vi "Process.vi"(8 "error in":errorcluster, 11 "Edit.Rect":refnum<class "Edit.Rect.lvclass">) -> (0 "error out":errorcluster, 3 "Edit.Rect out":refnum<class "Edit.Rect.lvclass">)   [LabVIEW 2019, in "Edit.Rect.lvclass"]
doc: "---------------------------------------------------------------\nJKI State Machine Objects™\nhttp://jki.net/state-machine-objects/\nCopyright (C) 2005-2015, JKI <info@jki.net>\nALL RIGHTS RESERVED"
uses:
  Edit.Rect.lvclass
  <vilib>/JKI/JKI SMO/SMO/SMO.lvclass
  <vilib>/JKI/JKI SMO/SMO/Typedefs/Parent Call--Enum.ctl
  Edit/Edit.lvclass
  subVIs/typedefs/Schedule Types/Schedule--Constant.ctl
  Settings/ObjectSettings/ObjectSettings.lvclass
  Settings/Setting Database/Setting Database.lvclass
  Settings/Rectangle Settings/Rectangle Settings.lvclass
  Settings/Setting Database/Typedefs/PrivateEvents--Setting Database.SetDefaultRectangle.ctl
  Settings/Setting Database/Typedefs/PrivateEvents--Setting Database.CopyActiveRectangleToAll.ctl
  C:/Users/Albro/Documents/GitHub/AFM-Lithography/lvsrc/Classes/Settings/ObjectSettings/ObjectSettings.lvclass
  C:/Program Files (x86)/National Instruments/LabVIEW 2019/vi.lib/JKI/JKI SMO/SMO/SMO.lvclass
  <vilib>/Utility/miscctls.llb/LVPointTypeDef.ctl
  Settings/Setting Database/Typedefs/PrivateEvents--Setting Database.Copy Settings To Group.ctl
panel:
  in  "Apply":bool
  out "Group String":string
  out "ID String":string
  in  "Apply All":bool
  in  "Speed Settings":bool
  in  "Voltage Settings":bool
  in  "Save Default":bool
  in  "Copy to All":bool
  in  "Fill Orientation":u16(ring) caption="Ring" items=["Horizontal", "Vertical"]
  in  "Enabled?":bool=TRUE
  in  "Direction":u16(ring) caption="Ring" items=["Forward", "Backward"]
  in  "Voltage Schedule":u16(ring) caption="Ring" items=["Constant", "Ramp", "Fn. Generator", "Formula"]
  in  "Speed Schedule":u16(ring) caption="Ring" items=["Constant", "Ramp", "Fn. Generator", "Formula"]
  in  "Set Resistance":T1(ring) caption="Enum"
  in  "Speed (um/s)":dbl caption="Numeric 2"
  in  "Voltage (V)":dbl caption="Numeric 2"
  in  "Fill Spacing":dbl caption="Numeric 2"
  # "For instructions on how to use the JKI State Machine Objects, examples and video tutorials, visit:\nhttp://jki.net/state-machine-objects/\n\nJKI State Machine Objects™\nhttp://jki.net/state-machine-objects/\nCopyright (C) 2005-2015, JKI <info@jki.net>\nALL RIGHTS RESERVED"
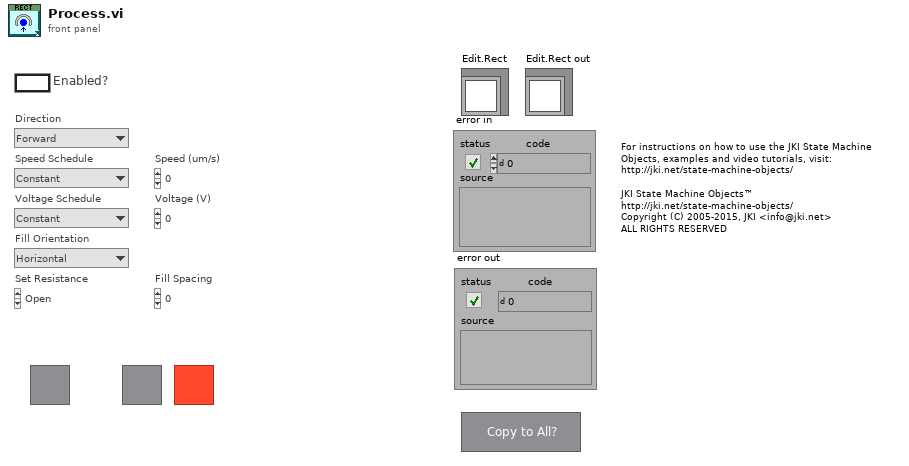
[diagram p1: front panel]
types:
  T1 = enum16{"Open", "Discharge Tip", "0 ohm", "100 kohm", "10 Mohm", "1 Gohm"}
  T2 = typedef "SMO.lvclass/Parent Call--Enum.ctl" = enum16{"Allows parent to run", "Does not request parent to run"}
  T3 = typedef "Schedule--Constant.ctl" = cluster{"Value":dbl}
  T4 = enum32{"invalid app kind", "Development System", "Run Time System", "Student Edition", "Embedded LabVIEW", "Evaluation", "Custom"}
  T5 = typedef "LVPointTypeDef.ctl" = cluster{"Horizontal":i16, "Vertical":i16}
  T6 = enum8{"Enabled", "Disabled", "Disabled and Grayed Out"}
  T7 = enum32{"Invalid", "Standard", "Closed", "Hidden", "Minimized", "Maximized"}
  T8 = enum32{"Bad", "Idle", "Run top level", "Running"}
  T9 = typedef "Setting Database.lvclass/PrivateEvents--Setting Database.Copy Settings To Group.ctl" = cluster{"Name":string, "Group":string}
  T10 = typedef "Setting Database.lvclass/PrivateEvents--Setting Database.SetDefaultRectangle.ctl" = bool
  T11 = typedef "Setting Database.lvclass/PrivateEvents--Setting Database.CopyActiveRectangleToAll.ctl" = bool
  T12 = typedef "Setting Database.lvclass/PublicEvents--Setting Database.NewActiveRectangle.ctl" = refnum<class "Rectangle Settings.lvclass">
  T13 = cluster{"Core":cluster{"Current VI Reference":refnum<vi>, "Close Panel on Exit?":bool, "error":errorcluster}, "Self":refnum<class "Edit.Rect.lvclass">, "SettingDB":refnum<class "Setting Database.lvclass">, "Rectangle Settings":refnum<class "Rectangle Settings.lvclass">}
  T14 = cluster{"Current VI Reference":refnum<vi>, "Close Panel on Exit?":bool, "error":errorcluster}
  T15 = enum16{"Always On", "Always Off", "Off While Running"}
  T16 = typedef "SMO.lvclass/Protected Events.ctl" = cluster{"StopProcesses":refnum<user-event>, "AbortProcesses":refnum<user-event>, "Config Changed":refnum<user-event>, "Dependency":refnum<user-event>}
  T17 = typedef "Setting Database.lvclass/PublicEvents--Cluster.ctl" = cluster{"NewActivePath":refnum<user-event>, "PathsUpdated":refnum<user-event>, "RectanglesUpdated":refnum<user-event>, "NewActiveRectangle":refnum<user-event>, "NewActiveFunnel":refnum<user-event>, "FunnelsUpdated":refnum<user-event>, "NewActiveDot":refnum<user-event>, "DotsUpdated":refnum<user-event>}
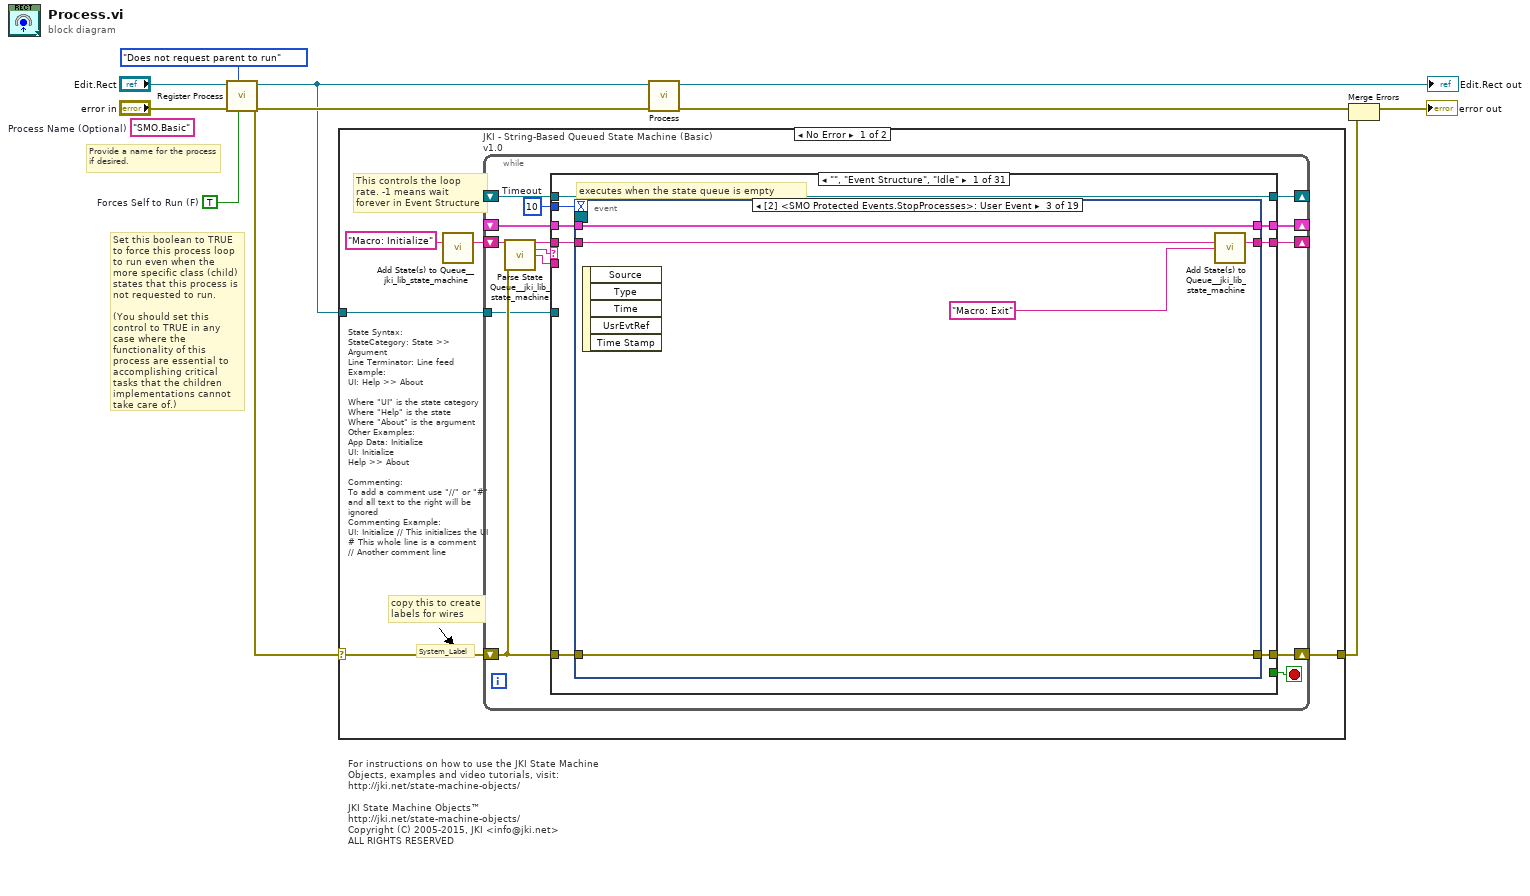
[diagram p0: block diagram]
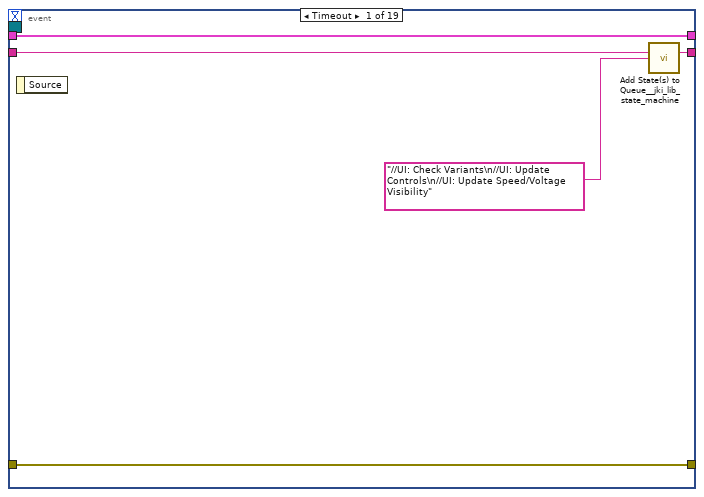
[diagram p2: hidden frame]
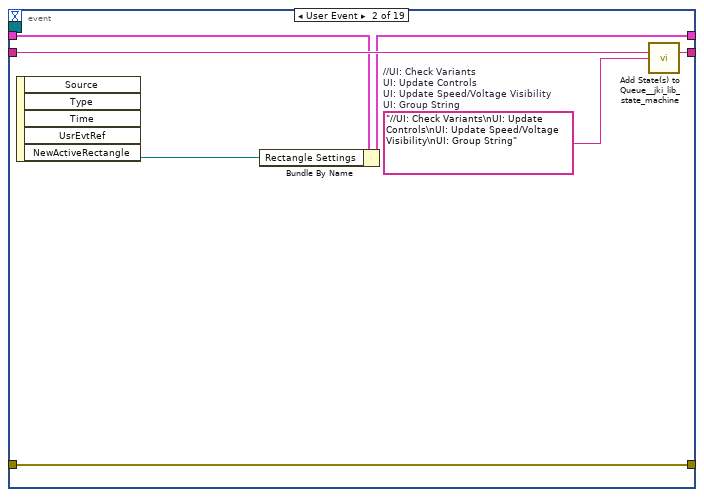
[diagram p3: hidden frame]
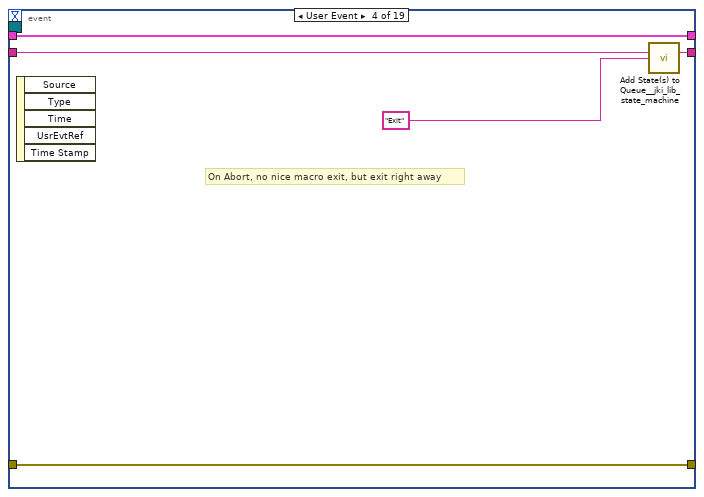
[diagram p4: hidden frame]
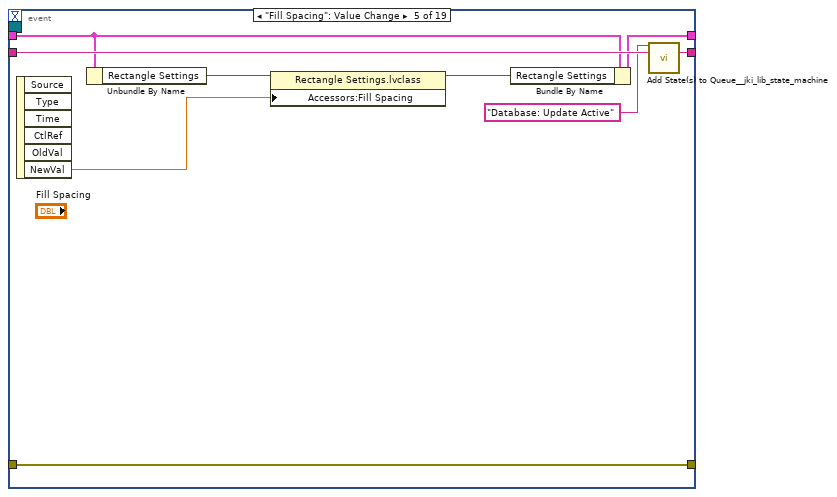
[diagram p5: hidden frame]
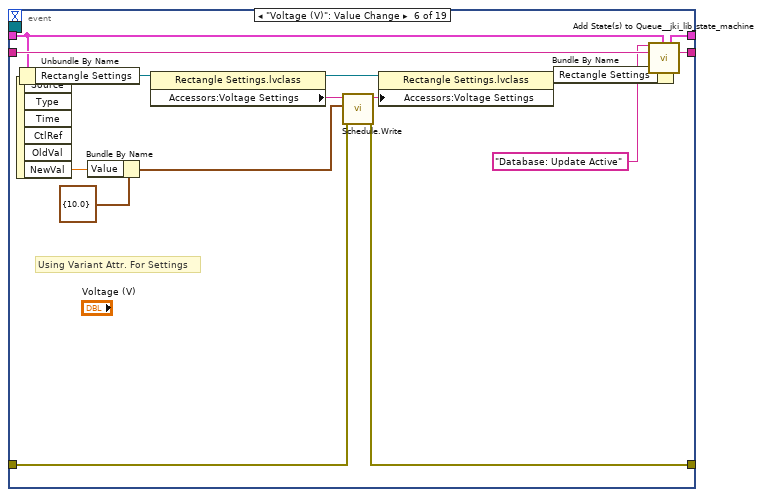
[diagram p6: hidden frame]
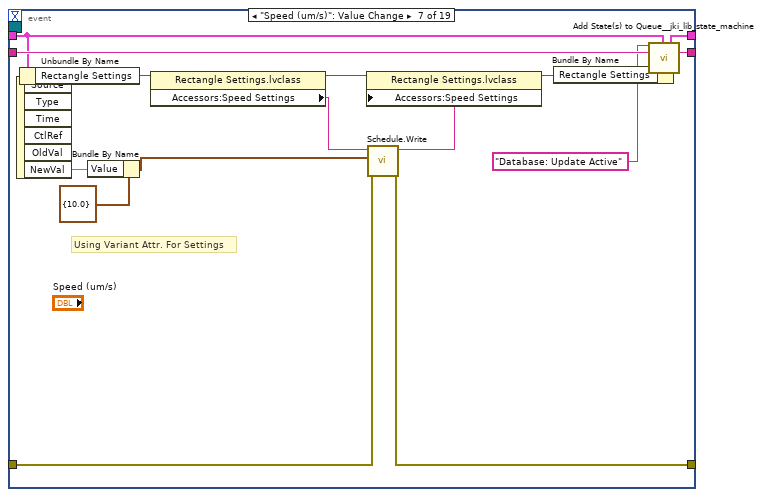
[diagram p7: hidden frame]
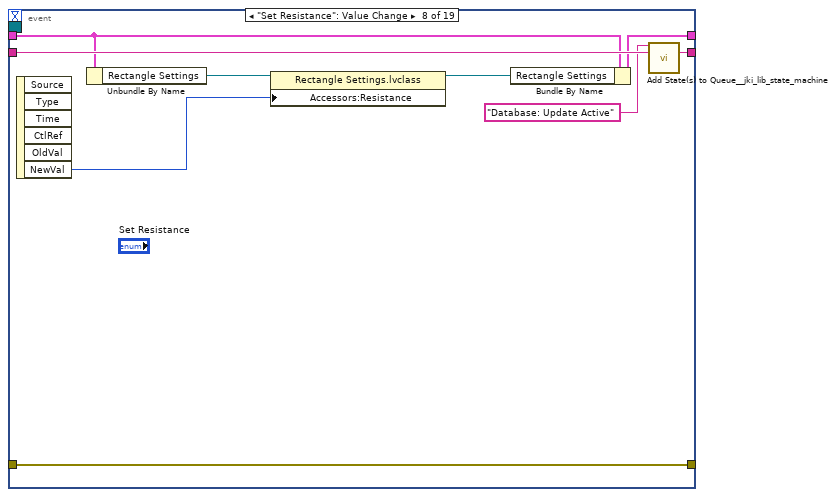
[diagram p8: hidden frame]
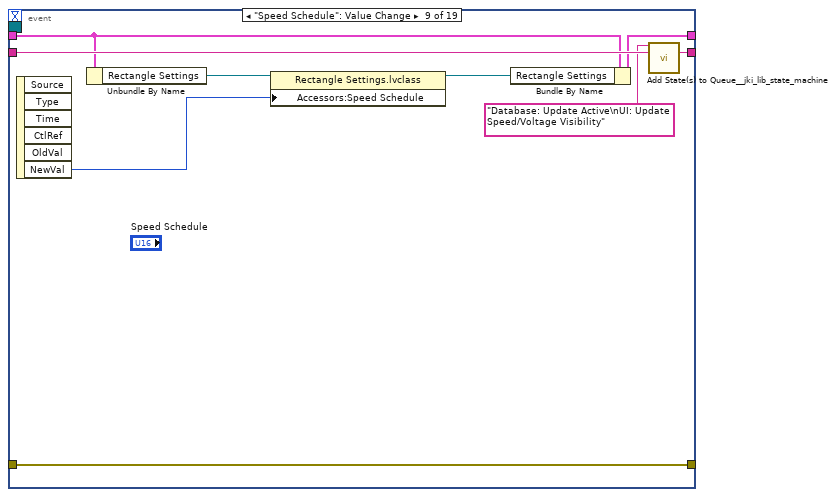
[diagram p9: hidden frame]
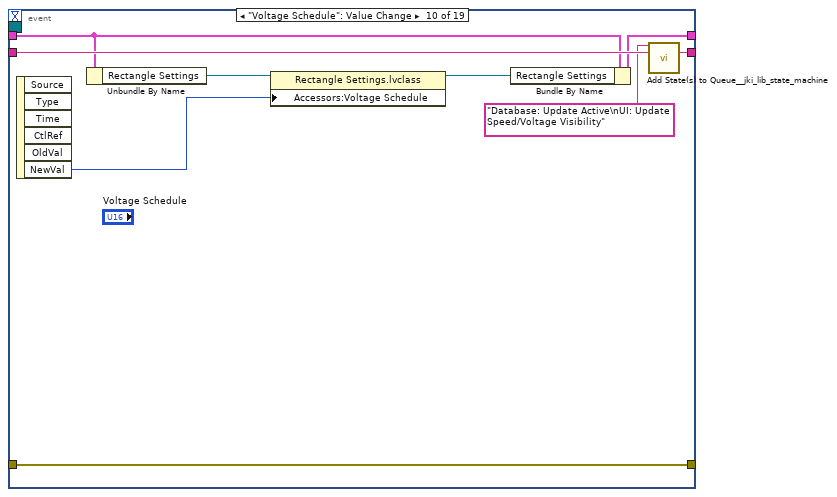
[diagram p10: hidden frame]
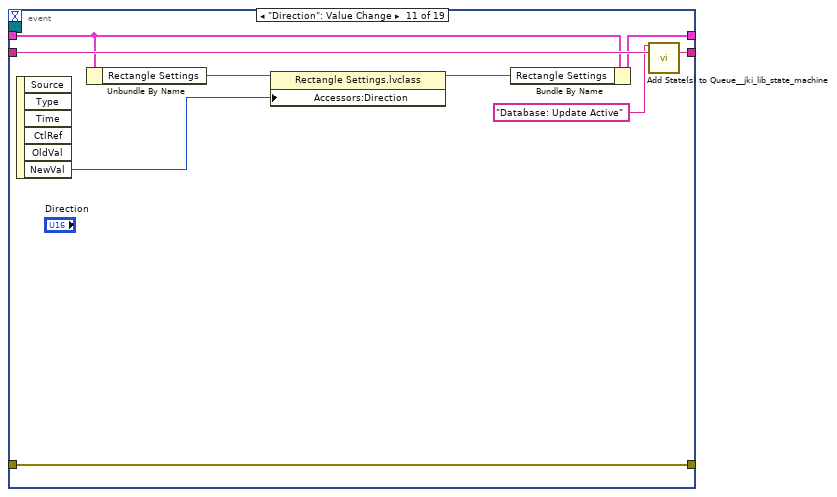
[diagram p11: hidden frame]
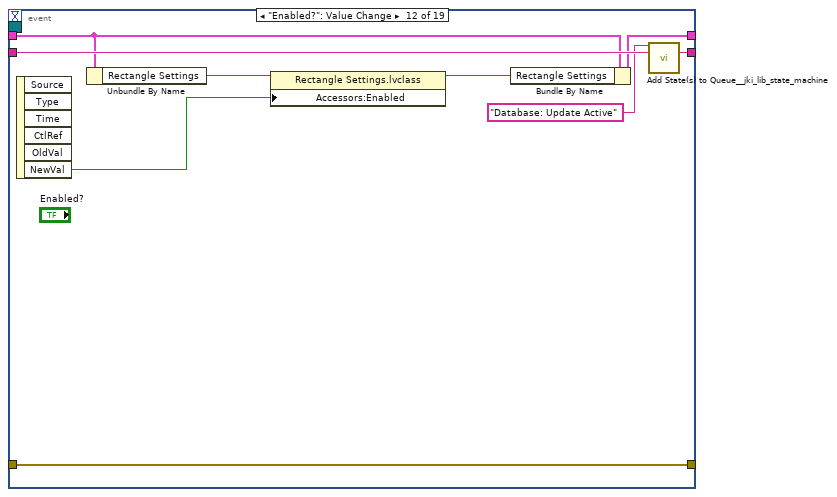
[diagram p12: hidden frame]
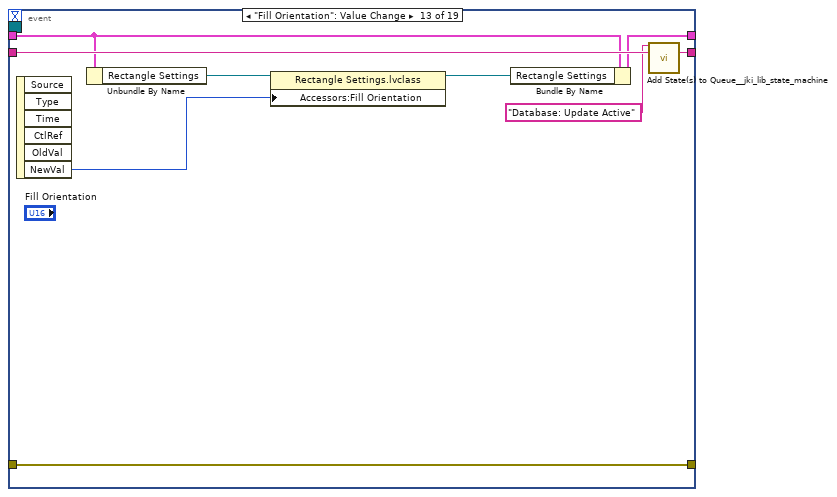
[diagram p13: hidden frame]
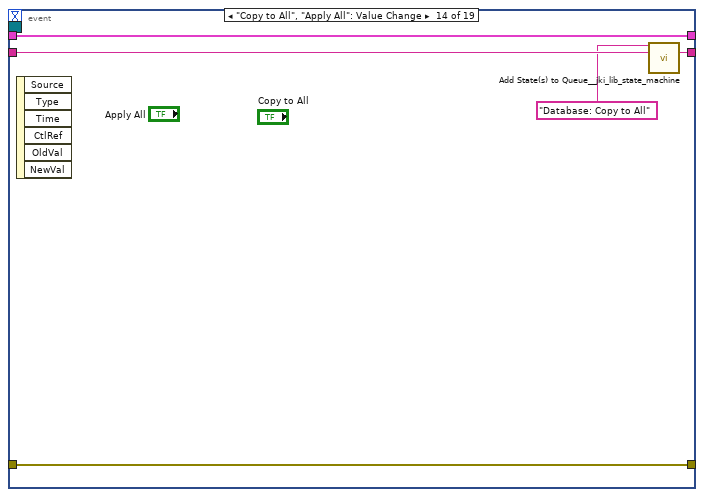
[diagram p14: hidden frame]
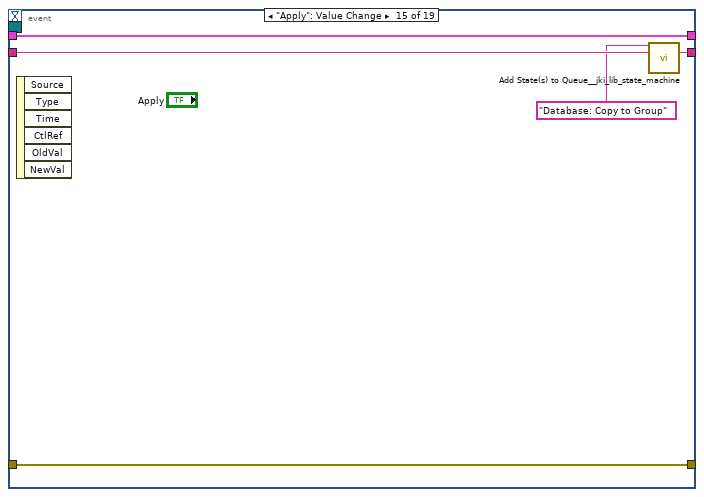
[diagram p15: hidden frame]
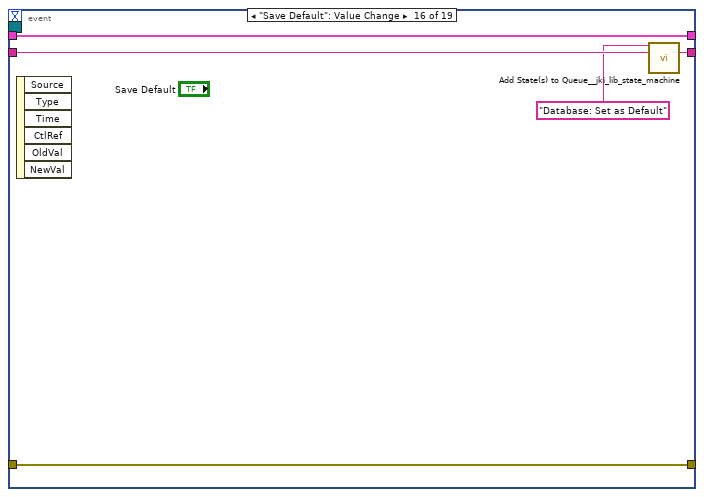
[diagram p16: hidden frame]
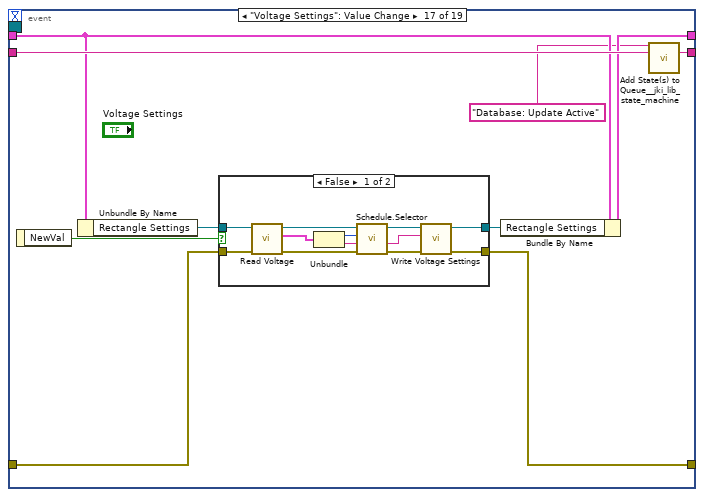
[diagram p17: hidden frame]
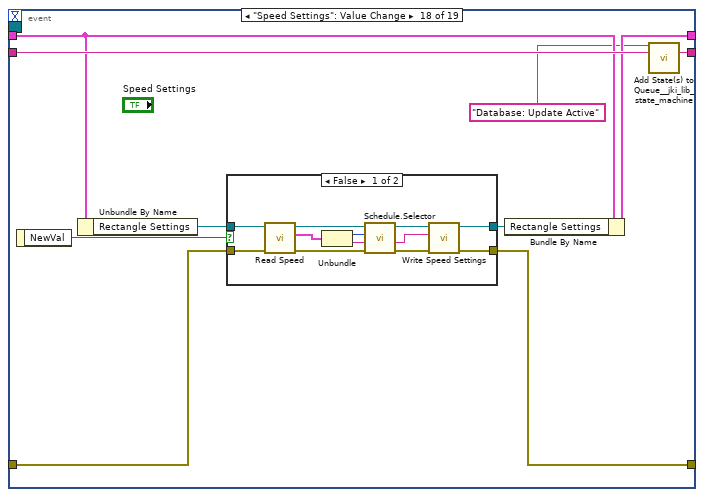
[diagram p19: hidden frame]
diagram:
  w2 = TRUE  # Forces Self to Run (F)
  (unwired) "SMO.Basic"  # Process Name (Optional)
  # "Provide a name for the process\nif desired."
  # "Set this boolean to TRUE to force this process loop to run even when the more specific class (child) states that this process is not requested to run.\n\n(You should set this control to TRUE in any case where the functionality of this process are essential to accomplishing critical tasks that the children implementations cannot take care of.)"
  # "For instructions on how to use the JKI State Machine Objects, examples and video tutorials, visit:\nhttp://jki.net/state-machine-objects/\n\nJKI State Machine Objects™\nhttp://jki.net/state-machine-objects/\nCopyright (C) 2005-2015, JKI <info@jki.net>\nALL RIGHTS RESERVED"
  n1 = call <vilib>:"Register Process.vi"("Forces Self to Run (F)"=w2, "Parent Call"=Parent_Call--Enum."Does not request parent to run", "error in (no error)"="error in", "SMO"="Edit.Rect") -> ("error out"=w7:errorcluster, "SMO out"=w1:refnum<class "Edit.Rect.lvclass">)  [unwired: 6 in]
  n2 = case shown="No Error" w7 {
    selector: w7 -> [w12 w582]
    tunnel: w1 -> [w13 _]
    tunnel: [w11 w582] -> w4
    frame No Error {
      # "State Syntax:\nStateCategory: State >> Argument\nLine Terminator: Line feed\nExample:\nUI: Help >> About\n\nWhere \"UI\" is the state category\nWhere \"Help\" is the state\nWhere \"About\" is the argument\nOther Examples:\nApp Data: Initialize\nUI: Initialize\nHelp >> About\n\nCommenting:\nTo add a comment use \"//\" or \"#\" and all text to the right will be ignored\nCommenting Example:\nUI: Initialize // This initializes the UI\n# This whole line is a comment\n// Another comment line"
      # "copy this to create labels for wires"
      # "This controls the loop rate. -1 means wait forever in Event Structure"
      # "System_Label"
      n3 = call <vilib>:"Add State(s) to Queue__jki_lib_state_machine.vi"("State(s) in (\"\")"="Macro: Initialize") -> ("States Out"=w15:string)  [unwired: 14 in]
      n4 = while "JKI - String-Based Queued State Machine (Basic) v1.0" {
        shift-right: [w22] -> _
        shift-left: _ -> [w21]
        shift-right: [w25] -> w11
        shift-left: w12 -> [w19]
        shift-right: [w24] -> _
        shift-left: w15 -> [w26]
        shift-right: [w18] -> _
        shift-left: _ -> [w17]
        tunnel: w13 -> [w16]
        stop <- w23 stop-if-true
        w20 = 10  # Timeout
        n5 = call <vilib>:"Parse State Queue__jki_lib_state_machine.vi"("State Queue"=w26, "Error In (no error)"=w19) -> ("Remaining States"=w28:string, "Current State"=w29:string, "Arguments"=w27:string)  [unwired: 11 in]
        n6 = case shown="\"\", \"Event Structure\", \"Idle\"" w29 {
          selector: w29 -> [_ _ w232 _ _ _ _ _ _ _ _ _ _ _ _ _ _ _ _ _ _ _ _ _ _ _ _ _ _ _ _]
          tunnel: w28 -> [w37 w226 w230 w251 w265 w271 w276 w288 w295 w300 w313 w328 w342 w366 w373 w392 w404 w436 w450 w464 w469 w480 w485 w498 w504 w509 w523 w533 w543 w553 w570]
          tunnel: w27 -> [_ _ _ _ _ _ _ _ _ _ _ _ _ _ w369 _ w397 _ _ _ _ _ _ _ _ _ _ _ _ _ _]
          tunnel: w21 -> [w35 w223 w231 w244 w253 w267 w273 _ w292 w297 w307 w321 w335 w360 w368 w390 w398 w433 w447 w452 w466 w470 w482 w494 w502 w505 w512 w529 w539 w549 w557]
          tunnel: [w34 w224 w235 w249 errorcluster {"status"=FALSE, "code"=0, "source"=""} ("error out") w266 w274 w279 w290 w298 w304 w325 w337 w364 w370 w383 w399 w434 w448 w462 w467 w472 w483 w493 w499 w507 w511 w526 w535 w546 w555] -> w25
          tunnel: w19 -> [w33 w224 w234 w249 w252 _ w274 w278 w291 w298 w302 w324 w336 w364 w371 w386 w400 w434 w448 w462 w467 w471 w483 w492 w499 w507 w510 w525 w534 w545 w554]
          tunnel: [w36 w225 w233 w250 w264 w270 w275 w287 w294 w299 w312 w327 w341 w365 w372 w391 w403 w435 w449 w463 w468 w479 w484 w497 w503 w508 w522 w532 w542 w552 w569] -> w24
          tunnel: [_ _ _ _ _ TRUE _ _ _ _ _ _ _ _ _ _ _ _ _ _ _ _ _ _ _ _ _ _ _ _ _] -> w23
          tunnel: [w32 w223 w231 w243 w254 w267 w273 w286 w292 w297 w307 w322 w335 w360 w368 w390 w398 w433 w447 w452 w466 w470 w482 w494 w502 w505 w513 w530 w540 w550 w556] -> w22
          tunnel: w20 -> [w31 _ _ _ _ _ _ _ _ _ _ _ _ _ _ _ _ _ _ _ _ _ _ _ _ _ _ _ _ _ _]
          tunnel: [w30 w222 w227 w239 w262 w268 w272 w284 w289 w296 w311 w323 w340 w361 w367 w378 w402 w432 w446 w461 w465 w478 w481 w496 w501 w506 w521 w531 w541 w551 w568] -> w18
          tunnel: w17 -> [w30 w222 w227 w239 w262 w268 w272 w284 w289 w296 w311 w323 w340 w361 w367 w378 w402 w432 w446 w461 w465 w478 w481 _ w501 w506 w521 w531 w541 w551 w568]
          tunnel: w16 -> [_ _ _ _ _ _ _ w277 _ _ _ _ _ _ _ _ _ _ _ _ _ _ _ _ _ _ _ _ _ _ _]
          frame "", "Event Structure", "Idle" {
            # "executes when the state queue is empty"
            n7 = event shown="[2] <SMO Protected Events.StopProcesses>: User Event" {
              selector: w30 -> [_ _ _ _ _ _ _ _ _ _ _ _ _ _ _ _ _ _ _]
              dyn-events: _ -> [_ _ _ _ _ _ _ _ _ _ _ _ _ _ _ _ _ _ _]
              timeout: w31 -> [_ _ _ _ _ _ _ _ _ _ _ _ _ _ _ _ _ _ _]
              tunnel: w37 -> [w42 w49 w54 w59 w68 w83 w98 w107 w116 w125 w134 w143 w152 w157 w162 w167 w177 w201 w221]
              tunnel: [w41 w48 w53 w58 w67 w82 w97 w106 w115 w124 w133 w142 w151 w156 w161 w166 w176 w200 w220] -> w36
              tunnel: w35 -> [w39 w45 w50 w55 w63 w79 w94 w102 w111 w120 w129 w138 w147 w155 w160 w165 w174 w198 w218]
              tunnel: [w40 w47 w52 w57 w66 w70 w86 w105 w114 w123 w132 w141 w150 w154 w159 w164 w171 w194 w219] -> w34
              tunnel: w33 -> [w40 w47 w52 w57 w66 w71 w84 w105 w114 w123 w132 w141 w150 w154 w159 w164 w170 w192 w219]
              tunnel: [w39 w46 w50 w55 w65 w81 w96 w104 w113 w122 w131 w140 w149 w155 w160 w165 w175 w199 w218] -> w32
              event Timeout {
                n8 = event-data() -> ()  [unwired: 1 in, 1 out]
                n9 = call <vilib>:"Add State(s) to Queue__jki_lib_state_machine.vi"("State(s) in (\"\")"=w42, "State(s) at Back (\"\")"="//UI: Check Variants\n//UI: Update Controls\n//UI: Update Speed/Voltage Visibility") -> ("States Out"=w41:string)  [unwired: 13 in]
              }
              event User Event {
                w43 = "//UI: Check Variants\nUI: Update Controls\nUI: Update Speed/Voltage Visibility\nUI: Group String"  # //UI: Check Variants UI: Update Controls UI: Update Speed/Voltage Visibility UI: Group String
                n10 = event-data() -> ("NewActiveRectangle"=w44:T12)  [unwired: 1 in, 4 out]
                n11 = Bundle By Name(cluster=w45, "Rectangle Settings"=w44) -> (w46:T13)
                n12 = call <vilib>:"Add State(s) to Queue__jki_lib_state_machine.vi"("State(s) in (\"\")"=w49, "State(s) at Back (\"\")"=w43) -> ("States Out"=w48:string)  [unwired: 13 in]
              }
              event User Event {
                n13 = event-data() -> ()  [unwired: 1 in, 5 out]
                n14 = call <vilib>:"Add State(s) to Queue__jki_lib_state_machine.vi"("State(s) in (\"\")"=w54, "State(s) at Back (\"\")"="Macro: Exit") -> ("States Out"=w53:string)  [unwired: 13 in]
              }
              event User Event {
                # "On Abort, no nice macro exit, but exit right away"
                n15 = event-data() -> ()  [unwired: 1 in, 5 out]
                n16 = call <vilib>:"Add State(s) to Queue__jki_lib_state_machine.vi"("State(s) in (\"\")"=w59, "State(s) at Back (\"\")"="Exit") -> ("States Out"=w58:string)  [unwired: 13 in]
              }
              event "Fill Spacing": Value Change {
                n17 = event-data() -> ("NewVal"=w61:dbl)  [unwired: 1 in, 5 out]
                n18 = Unbundle By Name(w63) -> ("Rectangle Settings"=w64:refnum<class "Rectangle Settings.lvclass">)
                n19 = property class="Rectangle Settings.lvclass"(reference=w64, "Accessors:Fill Spacing"=w61) -> (reference out=w62:refnum<class "Rectangle Settings.lvclass">)  [unwired: 1 in, 1 out]
                n20 = Bundle By Name(cluster=w63, "Rectangle Settings"=w62) -> (w65:T13)
                n21 = call <vilib>:"Add State(s) to Queue__jki_lib_state_machine.vi"("State(s) in Front (\"\")"="Database: Update Active", "State(s) in (\"\")"=w68) -> ("States Out"=w67:string)  [unwired: 13 in]
              }
              event "Voltage (V)": Value Change {
                # "Using Variant Attr. For Settings"
                n22 = event-data() -> ("NewVal"=w74:dbl)  [unwired: 1 in, 5 out]
                n23 = Unbundle By Name(w79) -> ("Rectangle Settings"=w80:refnum<class "Rectangle Settings.lvclass">)
                n24 = Bundle By Name(cluster=T3 {"Value"=10.0} ("Constant"), "Value"=w74) -> (w69:T3)
                n25 = property class="Rectangle Settings.lvclass"(reference=w80) -> (reference out=w78:refnum<class "Rectangle Settings.lvclass">, "Accessors:Voltage Settings"=w73:string)  [unwired: 1 in, 1 out]
                n26 = call "Schedule.Write.vi"("error in (no error)"=w71, "Data to Write"=w69, "Schedule <JSON> In"=w73) -> ("error out"=w70:errorcluster, "Schedule <JSON> Out"=w72:string)  [unwired: 7 in]
                n27 = property class="Rectangle Settings.lvclass"(reference=w78, "Accessors:Voltage Settings"=w72) -> (reference out=w76:refnum<class "Rectangle Settings.lvclass">)  [unwired: 1 in, 1 out]
                n28 = Bundle By Name(cluster=w79, "Rectangle Settings"=w76) -> (w81:T13)
                n29 = call <vilib>:"Add State(s) to Queue__jki_lib_state_machine.vi"("State(s) in Front (\"\")"="Database: Update Active", "State(s) in (\"\")"=w83) -> ("States Out"=w82:string)  [unwired: 13 in]
              }
              event "Speed (um/s)": Value Change {
                # "Using Variant Attr. For Settings"
                n30 = event-data() -> ("NewVal"=w89:dbl)  [unwired: 1 in, 5 out]
                n31 = Unbundle By Name(w94) -> ("Rectangle Settings"=w95:refnum<class "Rectangle Settings.lvclass">)
                n32 = Bundle By Name(cluster=T3 {"Value"=10.0} ("Constant"), "Value"=w89) -> (w85:T3)
                n33 = property class="Rectangle Settings.lvclass"(reference=w95) -> (reference out=w93:refnum<class "Rectangle Settings.lvclass">, "Accessors:Speed Settings"=w88:string)  [unwired: 1 in, 1 out]
                n34 = call "Schedule.Write.vi"("error in (no error)"=w84, "Data to Write"=w85, "Schedule <JSON> In"=w88) -> ("error out"=w86:errorcluster, "Schedule <JSON> Out"=w87:string)  [unwired: 7 in]
                n35 = property class="Rectangle Settings.lvclass"(reference=w93, "Accessors:Speed Settings"=w87) -> (reference out=w91:refnum<class "Rectangle Settings.lvclass">)  [unwired: 1 in, 1 out]
                n36 = Bundle By Name(cluster=w94, "Rectangle Settings"=w91) -> (w96:T13)
                n37 = call <vilib>:"Add State(s) to Queue__jki_lib_state_machine.vi"("State(s) in Front (\"\")"="Database: Update Active", "State(s) in (\"\")"=w98) -> ("States Out"=w97:string)  [unwired: 13 in]
              }
              event "Set Resistance": Value Change {
                n38 = event-data() -> ("NewVal"=w100:T1)  [unwired: 1 in, 5 out]
                n39 = Unbundle By Name(w102) -> ("Rectangle Settings"=w103:refnum<class "Rectangle Settings.lvclass">)
                n40 = property class="Rectangle Settings.lvclass"(reference=w103, "Accessors:Resistance"=w100) -> (reference out=w101:refnum<class "Rectangle Settings.lvclass">)  [unwired: 1 in, 1 out]
                n41 = Bundle By Name(cluster=w102, "Rectangle Settings"=w101) -> (w104:T13)
                n42 = call <vilib>:"Add State(s) to Queue__jki_lib_state_machine.vi"("State(s) in Front (\"\")"="Database: Update Active", "State(s) in (\"\")"=w107) -> ("States Out"=w106:string)  [unwired: 13 in]
              }
              event "Speed Schedule": Value Change {
                n43 = event-data() -> ("NewVal"=w109:u16)  [unwired: 1 in, 5 out]
                n44 = Unbundle By Name(w111) -> ("Rectangle Settings"=w112:refnum<class "Rectangle Settings.lvclass">)
                n45 = property class="Rectangle Settings.lvclass"(reference=w112, "Accessors:Speed Schedule"=w109) -> (reference out=w110:refnum<class "Rectangle Settings.lvclass">)  [unwired: 1 in, 1 out]
                n46 = Bundle By Name(cluster=w111, "Rectangle Settings"=w110) -> (w113:T13)
                n47 = call <vilib>:"Add State(s) to Queue__jki_lib_state_machine.vi"("State(s) in Front (\"\")"="Database: Update Active\nUI: Update Speed/Voltage Visibility", "State(s) in (\"\")"=w116) -> ("States Out"=w115:string)  [unwired: 13 in]
              }
              event "Voltage Schedule": Value Change {
                n48 = event-data() -> ("NewVal"=w118:u16)  [unwired: 1 in, 5 out]
                n49 = Unbundle By Name(w120) -> ("Rectangle Settings"=w121:refnum<class "Rectangle Settings.lvclass">)
                n50 = property class="Rectangle Settings.lvclass"(reference=w121, "Accessors:Voltage Schedule"=w118) -> (reference out=w119:refnum<class "Rectangle Settings.lvclass">)  [unwired: 1 in, 1 out]
                n51 = Bundle By Name(cluster=w120, "Rectangle Settings"=w119) -> (w122:T13)
                n52 = call <vilib>:"Add State(s) to Queue__jki_lib_state_machine.vi"("State(s) in Front (\"\")"="Database: Update Active\nUI: Update Speed/Voltage Visibility", "State(s) in (\"\")"=w125) -> ("States Out"=w124:string)  [unwired: 13 in]
              }
              event "Direction": Value Change {
                n53 = event-data() -> ("NewVal"=w127:u16)  [unwired: 1 in, 5 out]
                n54 = Unbundle By Name(w129) -> ("Rectangle Settings"=w130:refnum<class "Rectangle Settings.lvclass">)
                n55 = property class="Rectangle Settings.lvclass"(reference=w130, "Accessors:Direction"=w127) -> (reference out=w128:refnum<class "Rectangle Settings.lvclass">)  [unwired: 1 in, 1 out]
                n56 = Bundle By Name(cluster=w129, "Rectangle Settings"=w128) -> (w131:T13)
                n57 = call <vilib>:"Add State(s) to Queue__jki_lib_state_machine.vi"("State(s) in Front (\"\")"="Database: Update Active", "State(s) in (\"\")"=w134) -> ("States Out"=w133:string)  [unwired: 13 in]
              }
              event "Enabled?": Value Change {
                n58 = event-data() -> ("NewVal"=w136:bool)  [unwired: 1 in, 5 out]
                n59 = Unbundle By Name(w138) -> ("Rectangle Settings"=w139:refnum<class "Rectangle Settings.lvclass">)
                n60 = property class="Rectangle Settings.lvclass"(reference=w139, "Accessors:Enabled"=w136) -> (reference out=w137:refnum<class "Rectangle Settings.lvclass">)  [unwired: 1 in, 1 out]
                n61 = Bundle By Name(cluster=w138, "Rectangle Settings"=w137) -> (w140:T13)
                n62 = call <vilib>:"Add State(s) to Queue__jki_lib_state_machine.vi"("State(s) in Front (\"\")"="Database: Update Active", "State(s) in (\"\")"=w143) -> ("States Out"=w142:string)  [unwired: 13 in]
              }
              event "Fill Orientation": Value Change {
                n63 = event-data() -> ("NewVal"=w145:u16)  [unwired: 1 in, 5 out]
                n64 = Unbundle By Name(w147) -> ("Rectangle Settings"=w148:refnum<class "Rectangle Settings.lvclass">)
                n65 = property class="Rectangle Settings.lvclass"(reference=w148, "Accessors:Fill Orientation"=w145) -> (reference out=w146:refnum<class "Rectangle Settings.lvclass">)  [unwired: 1 in, 1 out]
                n66 = Bundle By Name(cluster=w147, "Rectangle Settings"=w146) -> (w149:T13)
                n67 = call <vilib>:"Add State(s) to Queue__jki_lib_state_machine.vi"("State(s) in Front (\"\")"="Database: Update Active", "State(s) in (\"\")"=w152) -> ("States Out"=w151:string)  [unwired: 13 in]
              }
              event "Copy to All", "Apply All": Value Change {
                n68 = event-data() -> ()  [unwired: 1 in, 6 out]
                n69 = call <vilib>:"Add State(s) to Queue__jki_lib_state_machine.vi"("State(s) in Front (\"\")"="Database: Copy to All", "State(s) in (\"\")"=w157) -> ("States Out"=w156:string)  [unwired: 13 in]
              }
              event "Apply": Value Change {
                n70 = event-data() -> ()  [unwired: 1 in, 6 out]
                n71 = call <vilib>:"Add State(s) to Queue__jki_lib_state_machine.vi"("State(s) in Front (\"\")"="Database: Copy to Group", "State(s) in (\"\")"=w162) -> ("States Out"=w161:string)  [unwired: 13 in]
              }
              event "Save Default": Value Change {
                n72 = event-data() -> ()  [unwired: 1 in, 6 out]
                n73 = call <vilib>:"Add State(s) to Queue__jki_lib_state_machine.vi"("State(s) in Front (\"\")"="Database: Set as Default", "State(s) in (\"\")"=w167) -> ("States Out"=w166:string)  [unwired: 13 in]
              }
              event "Voltage Settings": Value Change {
                n74 = event-data() -> ("NewVal"=w169:bool)  [unwired: 1 in]
                n75 = Unbundle By Name(w174) -> ("Rectangle Settings"=w172:refnum<class "Rectangle Settings.lvclass">)
                n76 = case shown="False" w169 {
                  tunnel: w172 -> [w189 w191]
                  tunnel: [w181 w191] -> w173
                  tunnel: w170 -> [w188 w190]
                  tunnel: [w178 w190] -> w171
                  frame False {
                    n77 = call "Read Voltage.vi"("error in (no error)"=w188, "ObjectSettings in"=w189) -> ("error out"=w186:errorcluster, "Voltage"=w185:cluster{"Schedule":u16, "Settings":string}, "ObjectSettings out"=w187:refnum<class "Rectangle Settings.lvclass">)  [unwired: 7 in]
                    n78 = Unbundle(w185) -> ("Schedule"=w184:u16, "Settings"=w183:string)
                    n79 = call-dynamic "Schedule.Selector.vi"("error in (no error)"=w186, "Settings In"=w183, "Schedule"=w184, "ObjectSettings in"=w187) -> ("error out"=w180:errorcluster, "Settings Out"=w179:string, "ObjectSettings out"=w182:refnum<class "Rectangle Settings.lvclass">)  [unwired: 5 in]
                    n80 = call "Write Voltage Settings.vi"("error in (no error)"=w180, "Settings"=w179, "ObjectSettings in"=w182) -> ("error out"=w178:errorcluster, "ObjectSettings out"=w181:refnum<class "Rectangle Settings.lvclass">)  [unwired: 7 in]
                  }
                  frame True {
                  }
                }
                n81 = Bundle By Name(cluster=w174, "Rectangle Settings"=w173) -> (w175:T13)
                n82 = call <vilib>:"Add State(s) to Queue__jki_lib_state_machine.vi"("State(s) in Front (\"\")"="Database: Update Active", "State(s) in (\"\")"=w177) -> ("States Out"=w176:string)  [unwired: 13 in]
              }
              event "Speed Settings": Value Change {
                n83 = event-data() -> ("NewVal"=w193:bool)  [unwired: 1 in]
                n84 = Unbundle By Name(w198) -> ("Rectangle Settings"=w196:refnum<class "Rectangle Settings.lvclass">)
                n85 = case shown="False" w193 {
                  tunnel: w196 -> [w211 w215]
                  tunnel: [w205 w215] -> w195
                  tunnel: w192 -> [w209 w214]
                  tunnel: [w204 w214] -> w194
                  frame False {
                    n86 = call "Read Speed.vi"("error in (no error)"=w209, "ObjectSettings in"=w211) -> ("error out"=w208:errorcluster, "Speed"=w207:cluster{"Schedule":u16, "Settings":string}, "ObjectSettings out"=w210:refnum<class "Rectangle Settings.lvclass">)  [unwired: 7 in]
                    n87 = Unbundle(w207) -> ("Schedule"=w213:u16, "Settings"=w212:string)
                    n88 = call-dynamic "Schedule.Selector.vi"("error in (no error)"=w208, "Settings In"=w212, "Schedule"=w213, "ObjectSettings in"=w210) -> ("error out"=w203:errorcluster, "Settings Out"=w202:string, "ObjectSettings out"=w206:refnum<class "Rectangle Settings.lvclass">)  [unwired: 5 in]
                    n89 = call "Write Speed Settings.vi"("error in (no error)"=w203, "Settings"=w202, "ObjectSettings in"=w206) -> ("error out"=w204:errorcluster, "ObjectSettings out"=w205:refnum<class "Rectangle Settings.lvclass">)  [unwired: 7 in]
                  }
                  frame True {
                  }
                }
                n90 = Bundle By Name(cluster=w198, "Rectangle Settings"=w195) -> (w199:T13)
                n91 = call <vilib>:"Add State(s) to Queue__jki_lib_state_machine.vi"("State(s) in Front (\"\")"="Database: Update Active", "State(s) in (\"\")"=w201) -> ("States Out"=w200:string)  [unwired: 13 in]
              }
              event Panel Close? {
                # "Discard the event because we'll close the front panel ourselves in Macro: Exit"
                # "Close Panel button (pressed) Event\n(this executes Macro: Exit to terminate the VI)"
                n92 = event-data() -> ()  [unwired: 1 in, 1 out]
                n93 = event-data("Discard?"=TRUE) -> ()  [unwired: 1 in, 1 out]
                n94 = call <vilib>:"Add State(s) to Queue__jki_lib_state_machine.vi"("State(s) in Front (\"\")"="Macro: Exit", "State(s) in (\"\")"=w221) -> ("States Out"=w220:string)  [unwired: 13 in]
              }
            }
          }
          frame "---------- Core ----------" {
            # "Do not put any code in this frame.\n(it is a separator no-op)"
            n95 = call <vilib>:"Add State(s) to Queue__jki_lib_state_machine.vi"("State(s) in (\"\")"=w226) -> ("States Out"=w225:string)  [unwired: 14 in]
          }
          frame Default {
            w238 = 42 items=["No error", "Argument error", "Memory is full", "Out of zone", "End of file", "File already open", "Generic file I/O error", "File not found", "File permission error", "Disk is full", "Duplicate path", "Too many files open", "System feature not enabled", "Resource file not found", "Cannot add resource", "Resource not found", "Image not found", "Image memory error", "Pen does not exist", "Config type invalid", "Config token not found", "Config parse error", "Config memory error", "Bad external code format", "Bad external code offset", "External code not present", "Null window", "Destroy window error", "Null menu", "Print aborted", "Bad print record", "Print driver error", "Windows error during printing", "Memory error during printing", "Print dialog error", "Generic print error", "Invalid device refnum", "Device not found", "Device parameter error", "Device unit error", "Cannot open device", "Device call aborted", "Generic error", "Cancelled by user", "Object ID too low", "Object ID too high", "Object not in heap", "Unknown heap", "Unknown object (invalid DefProc)", "Unknown object (DefProc not in table)", "Message out of range", "Invalid (null) method", "Unknown message", "Manager call not supported", "Bad address", "Network operation in progress", "Network operation timed out", "Connection is busy", "Network attribute not supported", "Network error", "Address in use", "System out of memory", "Connection aborted", "Connection refused", "Not connected", "Already connected", "Connection closed", "Initialization error (interapplication manager)", "Bad occurrence", "Wait on unbound occurrence handler", "Occurrence queue overflow", "Datalog type conflict", "Unused", "Unrecognized type (interapplication manager)", "Memory corrupt", "Failed to make temporary DLL", "Old CIN version", "Drag socket not found", "Failed to load drop-object", "Failed to register OLE object", "Failed to release OLE object", "Format specifier type mismatch", "Unknown format specifier", "Too few format specifiers", "Too many format specifiers", "Scan failed", "Newer CIN version", "Error converting to variant", "Runtime menu error", "Password tampered", "Variant attribute not found", "Incompatible variant data type", "Event data is not available", "Event Store is not present", "Occurrence is not found", "Event Queue is not created", "Event info is not available", "Refnum passed is NULL", "Error retrieving Class GUID", "Error retrieving CoClass GUID", "Error retrieving TypeLib GUID.", "Bad built application magic bytes.", "Specific driver is different from the specific driver associated with the Logical Name.", "There is no session opened to the class driver.", "Max Error", "MAX - Error with config objects", "MAX - Error loading configuration", "MAX - Group not supported"]
            # "Current State"
            # "Do not delete, rename, or modify this frame.\n(this is used to capture unhandled states and typos)"
            # "Handle mistyped state name (developer tool)"
            n96 = Format Into String(format string="Software Exception: Unhandled State \"%s\"." ("message"), error in=w234, w232) -> (resulting string=w237:string, error out=w236:errorcluster)  [unwired: 1 in]
            n97 = call <vilib>:"Error Cluster From Error Code.vi"("show call chain? (False)"=TRUE, "error in (no error)"=w236, "error message (\"\")"=w237, "error code (0)"=w238) -> ("error out"=w235:errorcluster)  [unwired: 5 in]
            n98 = call <vilib>:"Add State(s) to Queue__jki_lib_state_machine.vi"("State(s) in (\"\")"=w230) -> ("States Out"=w233:string)  [unwired: 14 in]
          }
          frame "Initialize Core Data" {
            # "exe?"
            # "If panel starts closed or is an EXE, then close it when we exit"
            # "Do not delete, rename, or modify this frame.\n(this is used to determine panel behavior on exit)"
            n99 = property class="VI"() -> ("Front Panel.Open"=w247:bool)  [unwired: 2 in, 2 out]
            n100 = property class="App"() -> ("App.Kind"=w246:T4)  [unwired: 2 in, 2 out]
            n101 = control-ref of="Current VI Reference"() -> (w248:refnum<vi>)
            n102 = Not(x=w247) -> (.not. x?=w242:bool)
            n103 = Equal?(x=w246, y=T4."Run Time System" ("Application:Kind")) -> (x = y?=w241:bool)
            n104 = Or(x=w242, y=w241) -> (x .or. y?=w245:bool)
            n105 = Bundle By Name(cluster=w244, "Core.Current VI Reference"=w248, "Core.Close Panel on Exit?"=w245) -> (w243:T13)
            n106 = call <vilib>:"Add State(s) to Queue__jki_lib_state_machine.vi"("State(s) in (\"\")"=w251) -> ("States Out"=w250:string)  [unwired: 14 in]
          }
          frame "Error Handler" {
            w256 = TRUE  # Stop on Unhandled Error (T)
            # "Overwrite this method to handle errors and pass to parent if not handled. Parent will fire a public event if the error is not handled up the chain of classes."
            # "Unhandled Error -- Display it"
            # "Handle any errors here.\nYou can also output any states to clean-up after errors occur"
            # "Clear error"
            n107 = Unbundle By Name(w253) -> ("Self"=w261:refnum<class "Edit.Rect.lvclass">)
            n108 = call-dynamic "Handle Error.vi"("Stop on Unhandled Error (T)"=w256, "error in"=w252, "SMO"=w261) -> ("handling error"=w257:errorcluster, "Unhandled error"=w260:errorcluster)  [unwired: 6 in, 1 out]
            n109 = Bundle By Name(cluster=w253, "Core.error"=w260) -> (w254:T13)
            n110 = Select(t="Exit", s=w257, f="") -> (s? t:f=w255:string)
            n111 = call <vilib>:"Add State(s) to Queue__jki_lib_state_machine.vi"("State(s) in Front (\"\")"=w255, "State(s) in (\"\")"=w265) -> ("States Out"=w264:string)  [unwired: 13 in]
          }
          frame "Exit" {
            # "Do not put any code in this frame.\n(No errors that occur here will be handled.)"
            n112 = Unbundle By Name(w267) -> ("Core.error"=w266:errorcluster)
            n113 = call <vilib>:"Add State(s) to Queue__jki_lib_state_machine.vi"("State(s) in (\"\")"=w271) -> ("States Out"=w270:string)  [unwired: 14 in]
          }
          frame "---------- Data ----------" {
            # "Do not put any code in this frame.\n(It is a separator no-op. You can make a copy of this frame to create a new Data frame)"
            n114 = call <vilib>:"Add State(s) to Queue__jki_lib_state_machine.vi"("State(s) in (\"\")"=w276) -> ("States Out"=w275:string)  [unwired: 14 in]
          }
          frame "Data: Initialize" {
            w281 = refnum<class "Edit.Rect.lvclass"> refnum  # Self
            w282 = refnum<class "Rectangle Settings.lvclass"> refnum  # Rectangle Settings
            w283 = refnum<class "Setting Database.lvclass"> refnum  # SettingDB
            w285 = T14 {"Current VI Reference"=refnum, "Close Panel on Exit?"=FALSE, "error"={"status"=FALSE, "code"=0, "source"=""}}  # Core
            # "Initialize the shift-register data, here.\n(data names are defined by what you wire into the bundle function)"
            n115 = Variant To Data(error in=w278, type=w281, Variant=w277) -> (data=w280:refnum<class "Edit.Rect.lvclass">, error out=w279:errorcluster)
            n116 = Bundle("Core"=w285, "Self"=w280, "SettingDB"=w283, "Rectangle Settings"=w282) -> (w286:T13)  [unwired: 1 in]
            n117 = call <vilib>:"Add State(s) to Queue__jki_lib_state_machine.vi"("State(s) in (\"\")"=w288) -> ("States Out"=w287:string)  [unwired: 14 in]
          }
          frame "Data: Cleanup" {
            # "Cleanup any data and references, here.\n(this is called automatically, by the Macro: Exit)"
            n118 = Unbundle By Name(w292) -> ("Core.Current VI Reference"=w293:refnum<vi>)
            n119 = Close Reference(reference=w293, error in (no error)=w291) -> (error out=w290:errorcluster)
            n120 = call <vilib>:"Add State(s) to Queue__jki_lib_state_machine.vi"("State(s) in (\"\")"=w295) -> ("States Out"=w294:string)  [unwired: 14 in]
          }
          frame "---------- UI ----------" {
            # "Do not put any code in this frame.\n(It is a separator no-op. You can make a copy of this frame to create a new UI frame)"
            n121 = call <vilib>:"Add State(s) to Queue__jki_lib_state_machine.vi"("State(s) in (\"\")"=w300) -> ("States Out"=w299:string)  [unwired: 14 in]
          }
          frame "UI: Group String" {
            # "Do not put any code in this frame.\n(It is a separator no-op. You can make a copy of this frame to create a new UI frame)"
            n122 = Unbundle By Name(w307) -> ("Rectangle Settings"=w308:refnum<class "Rectangle Settings.lvclass">)
            n123 = control-ref of="Apply"() -> (w301:refnum<vi>)
            n124 = call-dynamic "Read GUID.vi"("ObjectSettings in"=w308) -> ("GUID"=→"ID String":string)  [unwired: 8 in, 2 out]
            n125 = call-dynamic "Read Group.vi"("error in (no error)"=w302, "ObjectSettings in"=w308) -> ("error out"=w303:errorcluster, "Group"=w305:string)  [unwired: 7 in, 1 out]
            "Group String" <- w305
            n126 = Empty String/Path?(string/path=w305) -> (empty?=w310:bool)
            n127 = Not(x=w310) -> (.not. x?=w309:bool)
            n128 = property class="Bool"(reference=w301, error in=w303, "Visible"=w309) -> (error out=w304:errorcluster)  [unwired: 1 out]
            n129 = call <vilib>:"Add State(s) to Queue__jki_lib_state_machine.vi"("State(s) in (\"\")"=w313) -> ("States Out"=w312:string)  [unwired: 14 in]
          }
          frame "UI: Check Variants" {
            # "Do not put any code in this frame.\n(It is a separator no-op. You can make a copy of this frame to create a new UI frame)"
            n130 = Unbundle By Name(w321) -> ("Rectangle Settings"=w320:refnum<class "Rectangle Settings.lvclass">)
            n131 = property class="Rectangle Settings.lvclass"(reference=w320) -> (reference out=w319:refnum<class "Rectangle Settings.lvclass">, "Accessors:Voltage Settings"=w317:string, "Accessors:Speed Settings"=w315:string)  [unwired: 1 in, 1 out]
            n132 = call "Schedule.CheckVariantAttributes.vi"("error in (no error)"=w324, "Schedule <JSON> In"=w315) -> ("error out"=w326:errorcluster, "Schedule <JSON> Out"=w314:string)  [unwired: 8 in]
            n133 = call "Schedule.CheckVariantAttributes.vi"("error in (no error)"=w326, "Schedule <JSON> In"=w317) -> ("error out"=w325:errorcluster, "Schedule <JSON> Out"=w316:string)  [unwired: 8 in]
            n134 = property class="Rectangle Settings.lvclass"(reference=w319, "Accessors:Voltage Settings"=w316, "Accessors:Speed Settings"=w314) -> (reference out=w318:refnum<class "Rectangle Settings.lvclass">)  [unwired: 1 in, 1 out]
            n135 = Bundle By Name(cluster=w321, "Rectangle Settings"=w318) -> (w322:T13)
            n136 = call <vilib>:"Add State(s) to Queue__jki_lib_state_machine.vi"("State(s) in (\"\")"=w328) -> ("States Out"=w327:string)  [unwired: 14 in]
          }
          frame "UI: Initialize" {
            w330 = T15."Off While Running" ("Horizontal Scrollbar Visibility")
            # "Initialize the User Interface, here.\n(this is called automatically, by the Macro: Init)"
            n137 = Unbundle By Name(w335) -> ("Core.Current VI Reference"=w334:refnum<vi>)
            n138 = control-ref of="Speed Schedule"() -> (w339:refnum<vi>)
            n139 = property class="VI"(reference=w334) -> ("Panel"=w333:refnum<vi>)  [unwired: 1 in, 2 out]
            n140 = property class="Ring (strict)"(reference=w339, error in=w336, "DisabledEnum"=T6."Disabled and Grayed Out" ("Disabled")) -> (error out=w337:errorcluster)  [unwired: 1 out]
            n141 = property class="Pnl"(reference=w333) -> ("Panes[]"=w332:refnum<vi>[])  [unwired: 1 in, 2 out]
            n142 = Index Array(array=w332) -> (element=w331:refnum<vi>)  [unwired: 1 in]
            n143 = property class="Pane"(reference=w331, "HorizScrollbarVisibility"=w330, "VertScrollbarVisibility"=w330, "Origin"=T5 {"Horizontal"=0, "Vertical"=0}) -> ()  [unwired: 1 in, 2 out]
            n144 = call <vilib>:"Add State(s) to Queue__jki_lib_state_machine.vi"("State(s) in (\"\")"=w342) -> ("States Out"=w341:string)  [unwired: 14 in]
          }
          frame "UI: Update Controls" {
            w349 = T3 {"Value"=10.0} ("Constant")
            # "Using Variant Attr. For Settings"
            n145 = Unbundle By Name(w360) -> ("Rectangle Settings"=w359:refnum<class "Rectangle Settings.lvclass">)
            n146 = property class="Rectangle Settings.lvclass"(reference=w359) -> ("Accessors:Enabled"=w358:bool, "Accessors:Direction"=w357:u16, "Accessors:Fill Orientation"=w356:u16, "Accessors:Fill Spacing"=w355:dbl, "Accessors:Speed Schedule"=w354:u16, "Accessors:Voltage Schedule"=w353:u16, "Accessors:Resistance"=w352:T1, "Accessors:Speed Settings"=w346:string, "Accessors:Voltage Settings"=w344:string)  [unwired: 1 in, 2 out]
            n147 = local write "Enabled?"(w358) -> ()
            n148 = local write "Fill Orientation"(w356) -> ()
            n149 = local write "Speed Schedule"(w354) -> ()
            n150 = local write "Set Resistance"(w352) -> ()
            n151 = call "Schedule.CheckVariantAttributes.vi"("Schedule <JSON> In"=w346) -> ("Schedule <JSON> Out"=w345:string)  [unwired: 9 in, 1 out]
            n152 = call "Schedule.CheckVariantAttributes.vi"("Schedule <JSON> In"=w344) -> ("Schedule <JSON> Out"=w343:string)  [unwired: 9 in, 1 out]
            n153 = call "Schedule.Read.vi"("Data to Read"=w349, "Schedule <JSON> In"=w345) -> ("Data Out"=w351:variant)  [unwired: 7 in, 2 out]
            n154 = call "Schedule.Read.vi"("Data to Read"=w349, "Schedule <JSON> In"=w343) -> ("Data Out"=w348:variant)  [unwired: 7 in, 2 out]
            n155 = local write "Direction"(w357) -> ()
            n156 = local write "Voltage Schedule"(w353) -> ()
            n157 = local write "Fill Spacing"(w355) -> ()
            n158 = Variant To Data(type=w349, Variant=w351) -> (data=w350:T3)  [unwired: 1 in, 1 out]
            n159 = Variant To Data(type=w349, Variant=w348) -> (data=w347:T3)  [unwired: 1 in, 1 out]
            n160 = Unbundle(w350) -> ("Value"=w363:dbl)
            n161 = Unbundle(w347) -> ("Value"=w362:dbl)
            n162 = local write "Speed (um/s)"(w363) -> ()
            n163 = local write "Voltage (V)"(w362) -> ()
            n164 = call <vilib>:"Add State(s) to Queue__jki_lib_state_machine.vi"("State(s) in (\"\")"=w366) -> ("States Out"=w365:string)  [unwired: 14 in]
          }
          frame "UI: Cursor Set" {
            # "Argument"
            # "Set and Unset Cursor Busy.\n(Usage: \"UI: Cursor Set >> Busy|Idle\")"
            n165 = case shown="\"Idle\", Default" w369 {
              tunnel: w371 -> [w375 w377]
              tunnel: [w374 w376] -> w370
              frame "Idle", Default {
                n166 = call <vilib>:"Unset Busy.vi"("error in (no error)"=w375) -> ("error out"=w374:errorcluster)  [unwired: 10 in]
              }
              frame "Busy" {
                n167 = call <vilib>:"Set Busy.vi"("error in (no error)"=w377) -> ("error out"=w376:errorcluster)  [unwired: 9 in, 1 out]
              }
            }
            n168 = call <vilib>:"Add State(s) to Queue__jki_lib_state_machine.vi"("State(s) in (\"\")"=w373) -> ("States Out"=w372:string)  [unwired: 14 in]
          }
          frame "UI: Update Speed/Voltage Visibility" {
            n169 = local read "Voltage Schedule"() -> (w388:u16)
            n170 = local read "Speed Schedule"() -> (w389:u16)
            n171 = case shown="0" w388 {
              tunnel: [TRUE FALSE] -> w385
              frame 0 {
              }
              frame 1, Default {
              }
            }
            n172 = case shown="0" w389 {
              tunnel: [TRUE FALSE] -> w387
              frame 0 {
              }
              frame 1, Default {
              }
            }
            n173 = property on="Voltage (V)" class="DigNum (strict)"(error in=w386, "Visible"=w385) -> (error out=w380:errorcluster)  [unwired: 1 in, 1 out]
            n174 = Not(x=w385) -> (.not. x?=w381:bool)
            n175 = property on="Voltage Settings" class="Bool (strict)"(error in=w380, "Visible"=w381) -> (error out=w379:errorcluster)  [unwired: 1 in, 1 out]
            n176 = property on="Speed (um/s)" class="DigNum (strict)"(error in=w379, "Visible"=w387) -> (error out=w382:errorcluster)  [unwired: 1 in, 1 out]
            n177 = Not(x=w387) -> (.not. x?=w384:bool)
            n178 = property on="Speed Settings" class="Bool (strict)"(error in=w382, "Visible"=w384) -> (error out=w383:errorcluster)  [unwired: 1 in, 1 out]
            n179 = call <vilib>:"Add State(s) to Queue__jki_lib_state_machine.vi"("State(s) in (\"\")"=w392) -> ("States Out"=w391:string)  [unwired: 14 in]
          }
          frame "UI: Front Panel State" {
            # "Argument"
            # "Set Front Panel Open or Closed\n(Usage: \"UI: Front Panel State >> Open|Close\")"
            n180 = Unbundle By Name(w398) -> ("Core.Current VI Reference"=w401:refnum<vi>)
            n181 = disable-structure shown="Default" {
              disable-tunnel: w400 -> [w408 w431]
              disable-tunnel: [w407 w431] -> w399
              disable-tunnel: w401 -> [w406 _]
              disable-tunnel: w397 -> [w405 _]
              frame condition #0 (active) {
                n182 = case shown="\"Close\"" w405 {
                  tunnel: w408 -> [w412 w425]
                  tunnel: [w414 w426] -> w407
                  tunnel: w406 -> [w413 w423]
                  frame "Open", Default {
                    n183 = property class="VI"(reference=w413, error in=w412) -> (reference out=w410:refnum<vi>, error out=w411:errorcluster, "FP.State"=w409:T7)
                    n184 = case shown="\"Closed\"" w409 {
                      tunnel: [w417 w420] -> w414
                      tunnel: w411 -> [w416 w420]
                      tunnel: w410 -> [w415 _]
                      frame "Closed" {
                        n185 = invoke class="VI" method="FP.Open"(reference=w415, error in=w416, "Activate"=TRUE, "State"=T7."Standard") -> (error out=w417:errorcluster)  [unwired: 1 in, 4 out]
                      }
                      frame Default {
                      }
                    }
                  }
                  frame "Close" {
                    n186 = property class="VI"(reference=w423, error in=w425) -> (reference out=w422:refnum<vi>, error out=w424:errorcluster, "FP.State"=w421:T7)
                    n187 = case shown="Default" w421 {
                      tunnel: [w427 w430] -> w426
                      tunnel: w424 -> [w427 w429]
                      tunnel: w422 -> [_ w428]
                      frame "Invalid", "Closed" {
                      }
                      frame Default {
                        n188 = invoke class="VI" method="FP.Close"(reference=w428, error in=w429) -> (error out=w430:errorcluster)  [unwired: 1 in, 2 out]
                      }
                    }
                  }
                }
              }
              frame condition #1 {
              }
            }
            n189 = call <vilib>:"Add State(s) to Queue__jki_lib_state_machine.vi"("State(s) in (\"\")"=w404) -> ("States Out"=w403:string)  [unwired: 14 in]
          }
          frame "---------- Macro ----------" {
            # "Do not put any code in this frame.\n(It is a separator no-op. You can make a copy of this frame to create a new Macro frame)"
            n190 = call <vilib>:"Add State(s) to Queue__jki_lib_state_machine.vi"("State(s) in (\"\")"=w436) -> ("States Out"=w435:string)  [unwired: 14 in]
          }
          frame "Macro: Initialize" {
            w438 = "Process: Sync"
            (unwired) "Data: Initialize\nInitialize Core Data\nDatabase: Locate\nEvents: Register\nUI: Initialize\n//UI: Check Variants\n//UI: Update Controls\n//UI: Update Speed/Voltage Visibility\n//UI: Front Panel State >> Close"
            # "Initialization Macro\n(This is called once, when the VI starts)"
            n191 = control-ref of="This VI"() -> (w440:refnum<vi>)
            n192 = property class="VI"(reference=w440) -> ("Exec.State"=w439:T8)  [unwired: 1 in, 2 out]
            n193 = Equal?(x=w439, y=T8."Run top level") -> (x = y?=w444:bool)
            n194 = Select(t=w438, s=w444, f="") -> ()  [unwired: 1 out]
            n195 = call <vilib>:"Add State(s) to Queue__jki_lib_state_machine.vi"("State(s) in Front (\"\")"="Data: Initialize\nInitialize Core Data\nDatabase: Locate\nEvents: Register", "State(s) in (\"\")"=w438, "State(s) at Back (\"\")"="UI: Initialize\n//UI: Check Variants\n//UI: Update Controls\n//UI: Update Speed/Voltage Visibility\n//UI: Front Panel State >> Close") -> ("States Out"=w437:string)  [unwired: 12 in]
            n196 = call <vilib>:"Add State(s) to Queue__jki_lib_state_machine.vi"("State(s) in Front (\"\")"=w437, "State(s) in (\"\")"=w450) -> ("States Out"=w449:string)  [unwired: 13 in]
          }
          frame "Macro: Exit" {
            # "Exit Macro\n(This is called once, when the VI exits)"
            n197 = Unbundle By Name(w452) -> ("Core.Close Panel on Exit?"=w460:bool)
            n198 = Select(t="UI: Front Panel State >> Close", s=w460, f="") -> (s? t:f=w457:string)
            n199 = call <vilib>:"Add State(s) to Queue__jki_lib_state_machine.vi"("State(s) in Front (\"\")"="Data: Cleanup\nEvents: Unregister", "State(s) in (\"\")"="Process: Sync", "State(s) at Back (\"\")"="Exit") -> ("States Out"=w454:string)  [unwired: 12 in]
            n200 = call <vilib>:"Add State(s) to Queue__jki_lib_state_machine.vi"("State(s) in (\"\")"=w457, "State(s) at Back (\"\")"=w454) -> ("States Out"=w451:string)  [unwired: 13 in]
            n201 = call <vilib>:"Add State(s) to Queue__jki_lib_state_machine.vi"("State(s) in Front (\"\")"=w451, "State(s) in (\"\")"=w464) -> ("States Out"=w463:string)  [unwired: 13 in]
          }
          frame "---------- Process ----------" {
            # "Do not put any code in this frame.\n(It is a separator no-op. You can make a copy of this frame to create a new Macro frame)"
            n202 = call <vilib>:"Add State(s) to Queue__jki_lib_state_machine.vi"("State(s) in (\"\")"=w469) -> ("States Out"=w468:string)  [unwired: 14 in]
          }
          frame "Process: Sync" {
            # "Do not put any code in this frame.\n(It is a separator no-op. You can make a copy of this frame to create a new Macro frame)"
            n203 = Unbundle By Name(w470) -> ("Self"=w474:refnum<class "Edit.Rect.lvclass">)
            n204 = call <vilib>:"WaitOnProcessSync.vi"("error in (no error)"=w471, "SMO"=w474) -> ("error out"=w472:errorcluster, "Don't run?"=w477:bool)  [unwired: 7 in, 1 out]
            n205 = Select(t="Data: Cleanup\nEvents: Unregister\nExit", s=w477, f="") -> (s? t:f=w473:string)
            n206 = call <vilib>:"Add State(s) to Queue__jki_lib_state_machine.vi"("State(s) in Front (\"\")"=w473, "State(s) in (\"\")"=w480) -> ("States Out"=w479:string)  [unwired: 13 in]
          }
          frame "---------- Events ----------" {
            # "Do not put any code in this frame.\n(It is a separator no-op. You can make a copy of this frame to create a new UI frame)"
            n207 = call <vilib>:"Add State(s) to Queue__jki_lib_state_machine.vi"("State(s) in (\"\")"=w485) -> ("States Out"=w484:string)  [unwired: 14 in]
          }
          frame "Events: Register" {
            # "Do not put any code in this frame.\n(It is a separator no-op. You can make a copy of this frame to create a new UI frame)"
            n208 = Unbundle By Name(w494) -> ("SettingDB"=w491:refnum<class "Setting Database.lvclass">, "Self"=w488:refnum<class "Edit.Rect.lvclass">)
            n209 = call <vilib>:"GetProtectedEvents.vi"("SMO"=w488) -> ("error out"=w486:errorcluster, "SMO Protected Events"=w487:T16)  [unwired: 8 in, 1 out]
            n210 = call "Setting Database.GetPublicEvents.vi"("Setting Database"=w491) -> ("error out"=w489:errorcluster, "Public Events"=w490:T17)  [unwired: 8 in, 1 out]
            n211 = register-events(w490, w487) -> (reference out=w496:refnum<event-registration>, error out=w495:errorcluster)  [unwired: 2 in]
            n212 = Merge Errors(w492, w495, w489, w486) -> (w493:errorcluster)
            n213 = call <vilib>:"Add State(s) to Queue__jki_lib_state_machine.vi"("State(s) in (\"\")"=w498) -> ("States Out"=w497:string)  [unwired: 14 in]
          }
          frame "Events: Unregister" {
            # "Do not put any code in this frame.\n(It is a separator no-op. You can make a copy of this frame to create a new UI frame)"
            n214 = Unregister For Events(event registration refnum=w501, error in=w499) -> (error out=w500:errorcluster)
            n215 = call <vilib>:"Clear Errors.vi"("error in (no error)"=w500) -> ()  [unwired: 5 in, 2 out]
            n216 = call <vilib>:"Add State(s) to Queue__jki_lib_state_machine.vi"("State(s) in (\"\")"=w504) -> ("States Out"=w503:string)  [unwired: 14 in]
          }
          frame "---------- Database ----------" {
            n217 = call <vilib>:"Add State(s) to Queue__jki_lib_state_machine.vi"("State(s) in (\"\")"=w509) -> ("States Out"=w508:string)  [unwired: 14 in]
          }
          frame "Database: Copy to Group" {
            n218 = Unbundle By Name(w512) -> ("SettingDB"=w519:refnum<class "Setting Database.lvclass">, "Rectangle Settings"=w520:refnum<class "Rectangle Settings.lvclass">)
            n219 = call-dynamic "Read Group.vi"("ObjectSettings in"=w520) -> ("Group"=w516:string)  [unwired: 8 in, 2 out]
            n220 = Bundle By Name(cluster=T9 {"Name"="", "Group"=""} ("Copy Settings To Group"), "Group"=w516, "Name"="r") -> (w514:T9)
            n221 = call "Setting Database.CopySettingsToGroup.vi"("error in (no error)"=w510, "Copy Settings To Group"=w514, "Setting Database"=w519) -> ("error out"=w511:errorcluster, "Setting Database out"=w517:refnum<class "Setting Database.lvclass">)  [unwired: 7 in]
            n222 = Bundle By Name(cluster=w512, "SettingDB"=w517) -> (w513:T13)
            n223 = call <vilib>:"Add State(s) to Queue__jki_lib_state_machine.vi"("State(s) in (\"\")"=w523) -> ("States Out"=w522:string)  [unwired: 14 in]
          }
          frame "Database: Set as Default" {
            n224 = Unbundle By Name(w529) -> ("SettingDB"=w528:refnum<class "Setting Database.lvclass">)
            n225 = call "Setting Database.SetDefaultRectangle.vi"("error in (no error)"=w525, "SetDefaultRectangle"=T10 TRUE, "Setting Database"=w528) -> ("error out"=w526:errorcluster, "Setting Database out"=w527:refnum<class "Setting Database.lvclass">)  [unwired: 7 in]
            n226 = Bundle By Name(cluster=w529, "SettingDB"=w527) -> (w530:T13)
            n227 = call <vilib>:"Add State(s) to Queue__jki_lib_state_machine.vi"("State(s) in (\"\")"=w533) -> ("States Out"=w532:string)  [unwired: 14 in]
          }
          frame "Database: Update Active" {
            n228 = Unbundle By Name(w539) -> ("SettingDB"=w538:refnum<class "Setting Database.lvclass">, "Rectangle Settings"=w536:refnum<class "Rectangle Settings.lvclass">)
            n229 = call "Setting Database.UpdateActiveRectangle.vi"("error in (no error)"=w534, "UpdateActiveRectangle"=w536, "Setting Database"=w538) -> ("error out"=w535:errorcluster, "Setting Database"=w537:refnum<class "Setting Database.lvclass">)  [unwired: 7 in]
            n230 = Bundle By Name(cluster=w539, "SettingDB"=w537) -> (w540:T13)
            n231 = call <vilib>:"Add State(s) to Queue__jki_lib_state_machine.vi"("State(s) in (\"\")"=w543) -> ("States Out"=w542:string)  [unwired: 14 in]
          }
          frame "Database: Copy to All" {
            n232 = Unbundle By Name(w549) -> ("SettingDB"=w548:refnum<class "Setting Database.lvclass">)
            n233 = call "Setting Database.CopyActiveRectangleToAll.vi"("error in (no error)"=w545, "CopyActiveRectangleToAll"=T11 TRUE, "Setting Database"=w548) -> ("error out"=w546:errorcluster, "Setting Database out"=w547:refnum<class "Setting Database.lvclass">)  [unwired: 7 in]
            n234 = Bundle By Name(cluster=w549, "SettingDB"=w547) -> (w550:T13)
            n235 = call <vilib>:"Add State(s) to Queue__jki_lib_state_machine.vi"("State(s) in (\"\")"=w553) -> ("States Out"=w552:string)  [unwired: 14 in]
          }
          frame "Database: Locate" {
            # "#todo\nDecide what to do if not found..."
            n236 = Unbundle By Name(w557) -> ("Self"=w562:refnum<class "Edit.Rect.lvclass">, "SettingDB"=w565:refnum<class "Setting Database.lvclass">)
            n237 = call "Setting Database Name.vi"("error in (no error)"=w554) -> ("error out"=w559:errorcluster, "Name"=w558:string)  [unwired: 9 in]
            n238 = call <vilib>:"ListSharedResources.vi"("error in (no error)"=w559, "Filter (regex|name)"=w558, "SMO in"=w562) -> ("error out"=w560:errorcluster, "resources found?"=w563:bool, "Shared Resources"=w567:refnum<class "SMO.lvclass">[], "SMO out"=w561:refnum<class "Edit.Rect.lvclass">)  [unwired: 5 in]
            n239 = case shown="True" w563 {
              tunnel: w567 -> [_ w581]
              tunnel: [w572 w577] -> w566
              tunnel: w565 -> [w572 w579]
              tunnel: w561 -> [w573 w578]
              tunnel: [w573 w578] -> w564
              tunnel: w560 -> [w571 w574]
              tunnel: [w571 w575] -> w555
              frame False {
              }
              frame True {
                n240 = Index Array(array=w581, index=0) -> (element=w580:refnum<class "SMO.lvclass">)
                n241 = To More Specific Class(target class=w579, reference=w580, error in=w574) -> (specific class reference=w577:refnum<class "Setting Database.lvclass">, error out=w575:errorcluster)
              }
            }
            n242 = Bundle By Name(cluster=w557, "Self"=w564, "SettingDB"=w566) -> (w556:T13)
            n243 = call <vilib>:"Add State(s) to Queue__jki_lib_state_machine.vi"("State(s) in (\"\")"=w570) -> ("States Out"=w569:string)  [unwired: 14 in]
          }
        }
      }
    }
    frame Error {
    }
  }
  n244 = call-parent "Process.vi"("error in"=w7, "Edit"=w1) -> ("error out"=w5:errorcluster, "Edit out"=→"Edit.Rect out":refnum<class "Edit.Rect.lvclass">)  [unwired: 8 in]
  n245 = Merge Errors(w5, w4) -> (→"error out":errorcluster)
